vi "Joystick to Square.vi"(11 "Joystick Axis":dbl) -> (3 "Squared":dbl)   [LabVIEW 2014]
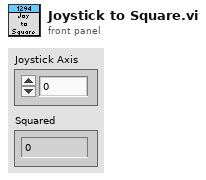
[diagram p1: front panel]
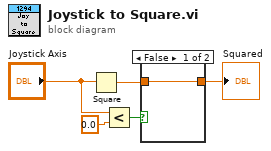
[diagram p0: block diagram]
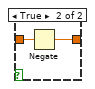
[diagram p2: hidden frame]
diagram:
  n1 = Square(x="Joystick Axis") -> (x^2=w3:dbl)
  n2 = Less?(x="Joystick Axis", y=0.0) -> (x < y?=w4:bool)
  n3 = case shown="False" w4 {
    tunnel: w3 -> [w6 w8]
    tunnel: [w6 w7] -> w1
    frame False {
    }
    frame True {
      n4 = Negate(x=w8) -> (-x=w7:dbl)
    }
  }
  "Squared" <- w1
